vi "UDP End Packet Test.vi"() -> ()   [LabVIEW 2014, in "ESP8266 WiFi Wrapper.lvlib"]
uses:
  ESP8266 WiFi Wrapper.lvlib
panel:
  out "Successful end packet?":bool
  out "Successful start packet?":bool
  out "Error Out":errorcluster
  in  "Error In":errorcluster
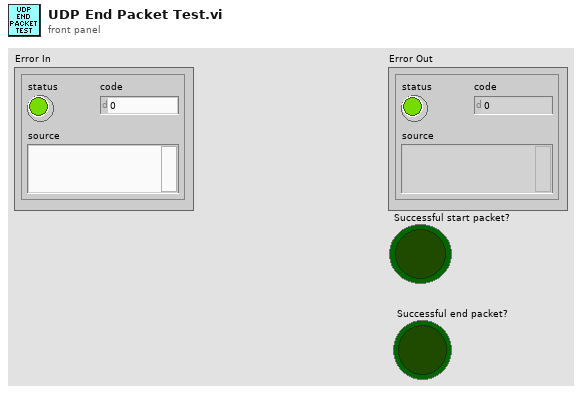
[diagram p1: front panel]
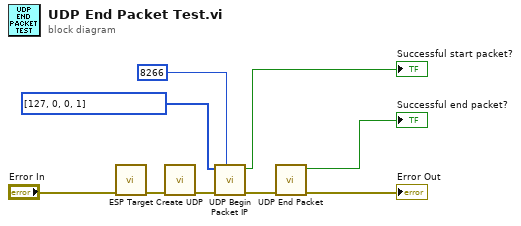
[diagram p0: block diagram]
diagram:
  n1 = call "ESP Target.vi"("Error In"="Error In") -> ("Error Out"=w8:errorcluster)  [unwired: 10 in]
  n2 = call "Create UDP.vi"("Error In"=w8) -> ("Error Out"=w7:errorcluster)  [unwired: 10 in]
  n3 = call <vilib>:"UDP Begin Packet IP.vi"("Port"=i16 8266, "Error In"=w7, "IP Address"=u8[] [127, 0, 0, 1]) -> ("Error Out"=w6:errorcluster, "Successful?"=→"Successful start packet?":bool)  [unwired: 7 in]
  n4 = call "UDP End Packet.vi"("Error In"=w6) -> ("Error Out"=→"Error Out":errorcluster, "Successful?"=→"Successful end packet?":bool)  [unwired: 9 in]
